vi "niRFUtil MT UTIL Fractional Resample Validate.vi"(0 "Waveform In":T1={"x0"=0.0, "dx"=1.0, "y"=[]} caption="input complex waveform" {"y" format="%.2f"; "dx" format="%^.2e"; "x0" format="%^.2e"}, 2 "Desired Sample Rate, Hz":dbl format="%.2f", 3 "Sample Phase Offset, sec":dbl format="%.2f") -> (15 "error out":errorcluster)   [LabVIEW 2015, in "niRFUtil.lvlib"]
doc: "Validates the inputs for the MT Fractional Resample VI."
uses:
  niRFUtil.lvlib
  Includes/niRFUtil INC Complex Waveform.ctl
  Includes/niRFUtil INC Complex Array.ctl
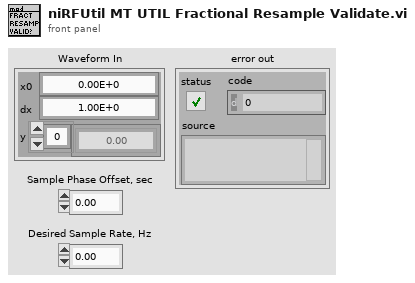
[diagram p1: front panel]
types:
  T1 = typedef "niRFUtil.lvlib/niRFUtil INC Complex Waveform.ctl" = cluster{"x0":dbl, "dx":dbl, "y":T2}
  T2 = typedef "niRFUtil.lvlib/niRFUtil INC Complex Array.ctl" = csg[]
  T3 = cluster{"status":bool, "code":i32, "name":string}[]
  T4 = cluster{"status":bool, "code":i32, "name":string}
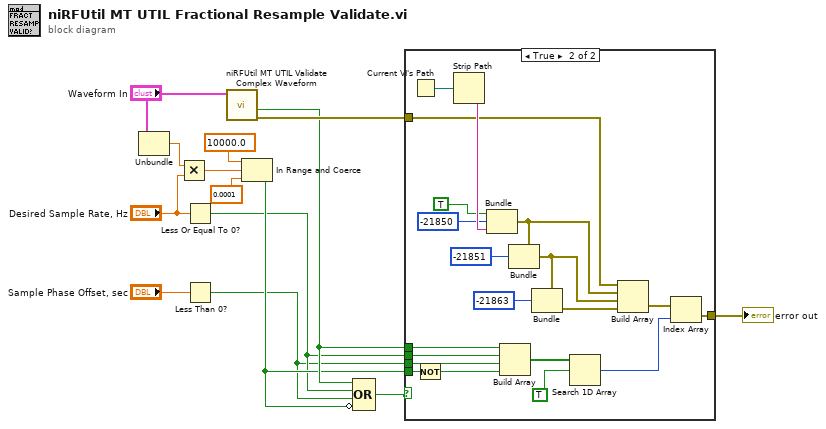
[diagram p0: block diagram]
diagram:
  n1 = Unbundle("Waveform In") -> ("dx"=w10:dbl)  [unwired: 2 out]
  n2 = Multiply(x=w10, y="Desired Sample Rate, Hz") -> (x*y=w8:dbl)
  n3 = Less Or Equal To 0?(x="Desired Sample Rate, Hz") -> (x <= 0?=w4:bool)
  n4 = Less Than 0?(x="Sample Phase Offset, sec") -> (x < 0?=w3:bool)
  n5 = call "niRFUtil MT UTIL Validate Complex Waveform.vi"("Waveform In"="Waveform In") -> ("error out"=w13:errorcluster, "error?"=w7:bool)  [unwired: 1 in, 8 out]
  n6 = In Range and Coerce(upper limit=10000.0, x=w8, lower limit=0.0001) -> (In Range?=w6:bool)  [unwired: 1 out]
  n7 = Compound Arithmetic op=OR(w7, w4, w3, invert w6) -> (w5:bool)
  n8 = case shown="True" w5 {
    tunnel: [_ w26] -> w14
    tunnel: w13 -> [_ w25]
    tunnel: w7 -> [_ w24]
    tunnel: w6 -> [_ w23]
    tunnel: w4 -> [_ w22]
    tunnel: w3 -> [_ w21]
    frame False {
    }
    frame True {
      n9 = Current VI's Path() -> (path=w27:path)
      n10 = Not(x=w23) -> (.not. x?=w15:bool)
      n11 = Strip Path(path=w27) -> (name=w34:string)  [unwired: 1 out]
      n12 = Bundle(TRUE, "code"=-21850, "name"=w34) -> (w19:cluster{bool, "code":i32, "name":string})  [unwired: 1 out]
      n13 = Build Array(w24, w22, w21, w15) -> (w30:bool[])
      n14 = Bundle(cluster=w19, "code"=-21851) -> (w17:cluster{bool, "code":i32, "name":string})  [unwired: 2 out]
      n15 = Bundle(cluster=w17, "code"=-21863) -> (w16:cluster{bool, "code":i32, "name":string})  [unwired: 2 out]
      n16 = Search 1D Array(1D array=w30, element=TRUE) -> (index of element=w28:i32)  [unwired: 1 out]
      n17 = Build Array(w25, w19, w17, w16) -> (w31:T3)
      n18 = Index Array(array=w31, index=w28) -> (element=w26:T4)
    }
  }
  "error out" <- w14
